vi "Read Key (U32).vi"(7 "section":string, 8 "error in (no error)":errorcluster, 9 "default value":u32, 10 "key":string, 11 "refnum":T1) -> (0 "error out":errorcluster, 1 "value":u32, 2 "found?":bool, 3 "refnum out":T1)   [LabVIEW 2010, in "NI_LVConfig.lvlib"]
doc: "Reads a value associated with a key in a specified section from the configuration data identified by <B>refnum</B>. If the key does not exist, the VI returns the default value. This VI supports multibyte characters in strings. Wire data to the <B>default value</B> input to determine the polymorphic instance to use or manually select the instance."
uses:
  NI_LVConfig.lvlib
  Config Data RefNum.ctl
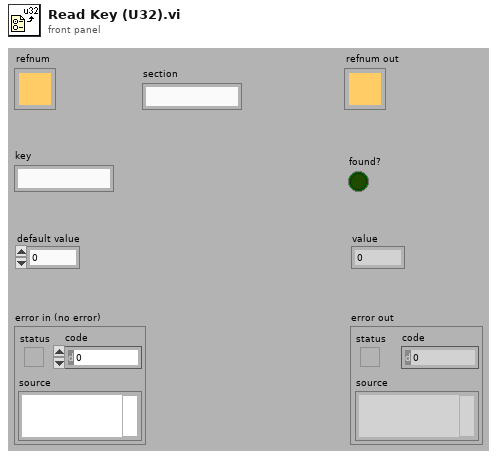
[diagram p1: front panel]
types:
  T1 = typedef "NI_LVConfig.lvlib/Config Data RefNum.ctl" = refnum<k1>
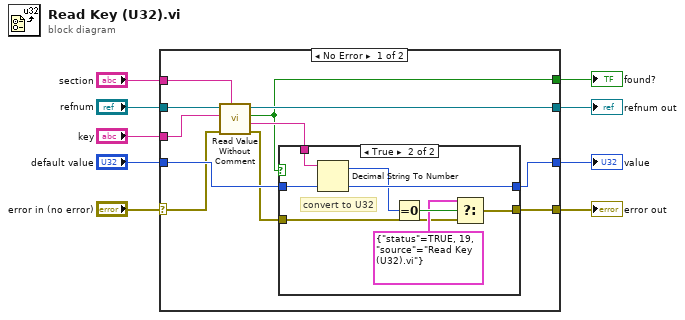
[diagram p0: block diagram]
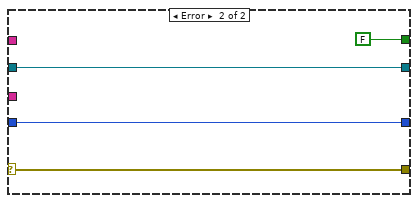
[diagram p3: hidden frame]
diagram:
  n1 = case shown="No Error" "error in (no error)" {
    selector: "error in (no error)" -> [w10 w34]
    tunnel: [w18 w34] -> w9
    tunnel: "section" -> [w17 _]
    tunnel: "key" -> [w12 _]
    tunnel: "default value" -> [w20 w33]
    tunnel: [w11 FALSE ("key exists?")] -> w6
    tunnel: [w19 w33] -> w4
    tunnel: [w16 w31] -> w3
    tunnel: "refnum" -> [w13 w31]
    frame No Error {
      n2 = call "Read Value Without Comment.vi"("section"=w17, "error in (no error)"=w10, "key"=w12, "refnum"=w13) -> ("error out"=w15:errorcluster, "value"=w14:string, "found?"=w11:bool, "refnum out"=w16:T1)  [unwired: 4 out]
      n3 = case shown="True" w11 {
        tunnel: [w22 w30] -> w19
        tunnel: w20 -> [w22 w29]
        tunnel: w15 -> [w21 w25]
        tunnel: [w21 w24] -> w18
        tunnel: w14 -> [_ w23]
        frame False {
        }
        frame True {
          # "convert to U32"
          n4 = Decimal String To Number(string=w23, default (0L)=w29) -> (offset past number=w26:i32, number=w30:u32)  [unwired: 1 out]
          n5 = Equal To 0?(x=w26) -> (x = 0?=w28:bool)
          n6 = Select(t=cluster{"status":bool, u16, "source":string} {"status"=TRUE, 19, "source"="Read Key (U32).vi"} ("f"), s=w28, f=w25) -> (s? t:f=w24:errorcluster)
        }
      }
    }
    frame Error {
    }
  }
  "error out" <- w9
  "found?" <- w6
  "value" <- w4
  "refnum out" <- w3
